vi "van der Pauw calc (2).vi"(2 "horizontal resistance":dbl, 3 "vertical resistance":dbl) -> (1 "Sheet resistance":dbl)   [LabVIEW 2019]
panel:
  out "N":i32
  out "ms counter":i32
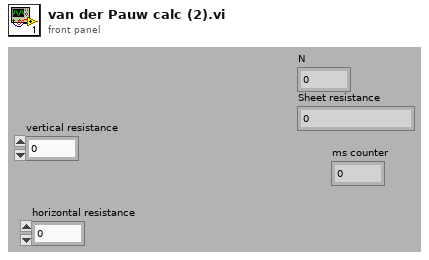
[diagram p1: front panel]
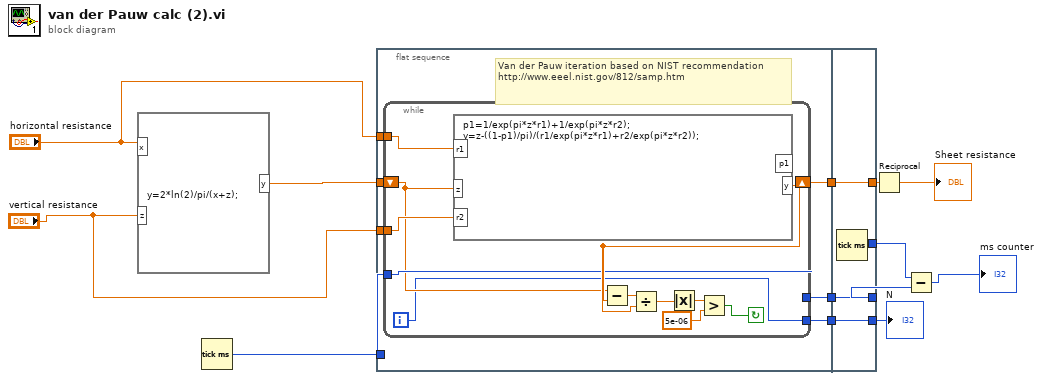
[diagram p0: block diagram]
diagram:
  n1 = formula code="y=2*ln(2)/pi/(x+z);"("x"="horizontal resistance", "z"="vertical resistance") -> ("y"=w13:dbl)
  n2 = Tick Count (ms)() -> (millisecond timer value=w6:u32)
  n3 = flat-sequence {
    tunnel: w13 -> [w20]
    tunnel: "horizontal resistance" -> [w19]
    tunnel: "vertical resistance" -> [w18]
    tunnel: w6 -> [w15]
    tunnel: [w17] -> w5
    tunnel: [w16] -> w4
    tunnel: [w14] -> w2
    tunnel: [w34] -> w8
    tunnel: [w35] -> w10
    tunnel: w5 -> [w35]
    tunnel: w4 -> [w34]
    tunnel: [w33] -> w3
    tunnel: w2 -> [w32]
    tunnel: [w32] -> w1
    frame #0 {
      # "Van der Pauw iteration based on NIST recommendation\nhttp://www.eeel.nist.gov/812/samp.htm"
      n4 = while {
        tunnel: w19 -> [w31]
        tunnel: w18 -> [w30]
        shift-right: [w28] -> w17
        shift-left: w20 -> [w22]
        tunnel: w15 -> [w23]
        tunnel: [w23] -> w16
        tunnel: [w21] -> w14
        i -> [w21]
        stop <- w25 continue-if-true
        n5 = formula code="p1=1/exp(pi*z*r1)+1/exp(pi*z*r2);\ny=z-((1-p1)/pi)/(r1/exp(pi*z*r1)+r2/exp(pi*z*r2));"("r1"=w31, "r2"=w30, "z"=w22) -> ("y"=w28:dbl)  [unwired: 1 out]
        n6 = Subtract(x=w22, y=w28) -> (x-y=w29:dbl)
        n7 = Divide(x=w29, y=w28) -> (x/y=w27:dbl)
        n8 = Absolute Value(x=w27) -> (abs(x)=w24:dbl)
        n9 = Greater?(x=w24, y=5e-06) -> (0:w25:bool)
      }
    }
    frame #1 {
      n10 = Tick Count (ms)() -> (millisecond timer value=w33:u32)
    }
  }
  n11 = Reciprocal(x=w10) -> (1/x=→"Sheet resistance":dbl)
  n12 = Subtract(x=w3, y=w8) -> (x-y=→"ms counter":u32)
  "N" <- w1
